vi "initialise_framescan.vi"(8 "error in (no error)":errorcluster) -> (0 "error out":errorcluster, 1 "config cluster":T1={"DDS board initialization parameters"={"Bypass PLL"=FALSE, "PLL Range"=TRUE, "Update Clock"=FALSE, "Triangle "=FALSE, "SDO Active"=FALSE, "LSB First"=FALSE, "OSK Int"=FALSE, "Output Shaped Keying Enable"=TRUE, "Bypass Sinc"=FALSE, "Digital Part"=TRUE, "OutPut DAC"=TRUE, "Control DAC"=TRUE, "Comparator"=FALSE, "Modus"=0, "Multiplier Value"=15}, "OSK select"=TRUE, "inverse?"="normal", "AOD equilibration time"=0.0, "AOD amplitude"=0, "AOD center frequency"=0.0, "AOD Bandwidth"=0.0} {"DDS board initialization parameters"."Modus" scale=0.0..4.0}, 2 "FPGA VI Reference Out":T3, 3 "network streaming queues out":T4)   [LabVIEW 2010]
uses:
  network_streaming_queues_cluster.ctl
  FPGAWrapperMH120124FrameScan_PXI7813R/settings_cluster_framescan.ctl
  common_typedefs/channels_cluster.ctl
  fpgaVIsAndControls/DDS_board_init_cluster.ctl
  fpgaVIsAndControls/gate_cluster.ctl
  common_typedefs/gate_parameters_cluster.ctl
  FPGAWrapperMH120124FrameScan_PXI7813R/configuration_cluster_framescan.ctl
  FPGAWrapperMH120124RAPS_PXI7813R/settings_cluster_raps.ctl
  fpgaVIsAndControls/ellipsoid_parameters_cluster.ctl
  FPGAWrapperMH120124RAPS_PXI7813R/configuration_cluster_raps.ctl
  FPGAWrapperMH120124FrameScan_PXI7813R/FPGA_framescan_reference.ctl
  fpgaVIsAndControls/inverse_enum.ctl
  command_enum.ctl
  <vilib>/userDefined/High Color/nirio_resource_hc.ctl
  <vilib>/rvi/interface/nirviOpenFPGA/nirviOpenFPGA.xnode
  FPGA Bitfiles/FPGA_frame.lvbitx
  <vilib>/rvi/ClientSDK/nirviWhatTheDeviceIsDoing.ctl
  <vilib>/rvi/interface/nirviMethod/nirviMethod.xnode
  <vilib>/rvi/interface/nirviReadWriteControl/nirviReadWriteControl.xnode
  <vilib>/rvi/interface/common/niFpgaNodeNameForErrorReporting.ctl
  <vilib>/rvi/errors/niLvFpgaWhatHappensToTopLevelVI.ctl
  <vilib>/FPGAPlugInAG/PXI-7813R/niLvFpga_Open_PXI-7813R.vi
  <vilib>/rvi/interface/common/dynamic/niFpgaDynamicAddResources.vi
  <vilib>/FPGAPlugInAG/Dynamic/niLvFpga_Reset_Dynamic.vi
  <vilib>/Utility/error.llb/Error Cluster From Error Code.vi
  <vilib>/rvi/errors/niLvFpgaAdjustHostInterfaceError.vi
  NiFpgaLv.dll
panel:
  # "FSK"
  # "Ramped"
  # "FSK"
  # "Chirp Modus"
  # "Unramped"
  # "BPSK"
  # "Single Tone"
  # "FSK"
  # "Ramped"
  # "FSK"
  # "Chirp Modus"
  # "Unramped"
  # "BPSK"
  # "Single Tone"
  # "FSK"
  # "Ramped"
  # "FSK"
  # "Chirp Modus"
  # "Unramped"
  # "BPSK"
  # "Single Tone"
  # "FSK"
  # "Ramped"
  # "FSK"
  # "Chirp Modus"
  # "Unramped"
  # "BPSK"
  # "Single Tone"
  # "FSK"
  # "Ramped"
  # "FSK"
  # "Chirp Modus"
  # "Unramped"
  # "BPSK"
  # "Single Tone"
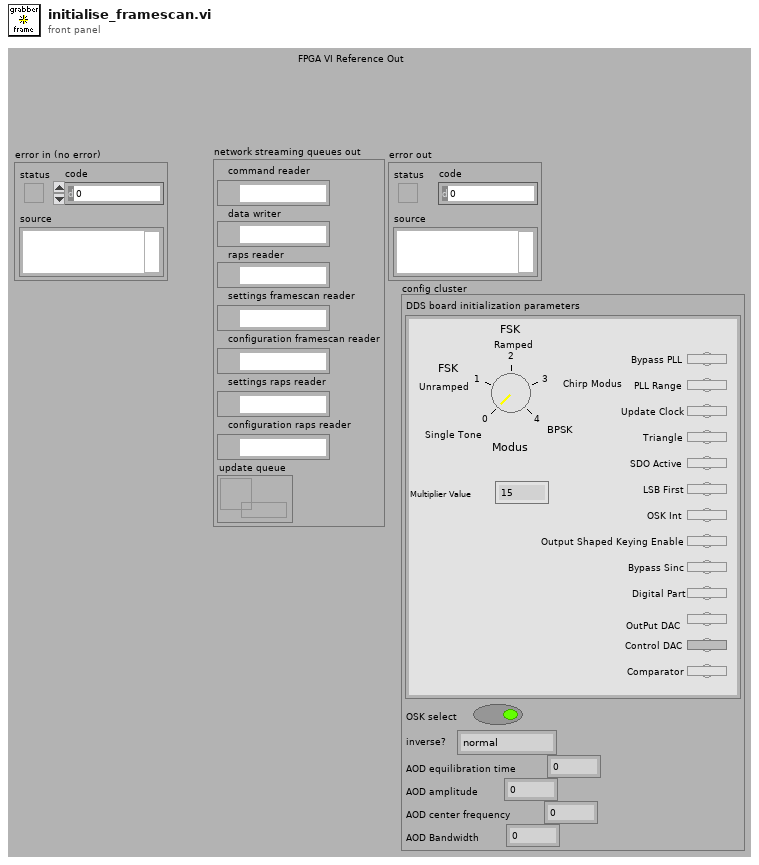
[diagram p1: front panel]
types:
  T1 = typedef "configuration_cluster_framescan.ctl" = cluster{"DDS board initialization parameters":T2, "OSK select":bool, "inverse?":string, "AOD equilibration time":dbl, "AOD amplitude":u16, "AOD center frequency":dbl, "AOD Bandwidth":dbl}
  T2 = typedef "DDS_board_init_cluster.ctl" = cluster{"Bypass PLL":bool, "PLL Range":bool, "Update Clock":bool, "Triangle ":bool, "SDO Active":bool, "LSB First":bool, "OSK Int":bool, "Output Shaped Keying Enable":bool, "Bypass Sinc":bool, "Digital Part":bool, "OutPut DAC":bool, "Control DAC":bool, "Comparator":bool, "Modus":u8, "Multiplier Value":u8}
  T3 = typedef "FPGA_framescan_reference.ctl" = refnum<k20>
  T4 = typedef "network_streaming_queues_cluster.ctl" = cluster{"command reader":refnum<k21>, "data writer":refnum<k21>, "raps reader":refnum<k21>, "settings framescan reader":refnum<k21>, "configuration framescan reader":refnum<k21>, "settings raps reader":refnum<k21>, "configuration raps reader":refnum<k21>, "update queue":refnum<queue>}
  T5 = typedef "inverse_enum.ctl" = enum16{"normal", "x inversed", "y inversed", "x & y inversed"}
  T6 = typedef "command_enum.ctl" = enum8{"NULL", "update", "start", "stop", "reset", "shut-down"}
  T7 = enum32{"Invalid", "Standard", "Closed", "Hidden", "Minimized", "Maximized"}
  T8 = typedef "settings_cluster_framescan.ctl" = cluster{"number of pixels":i32, "iterations per pixel":i32, "maximum bit-depth":i8, "AOD center freq. (Hz)":dbl, "AOD bandwidth freq. (Hz)":dbl, "AOD amplitude":dbl, "pixel dwell time":dbl, "AOD equilibration time":dbl, "x resolution":i32, "y resolution":i32, "z angle (rotation angle, phi)":dbl, "x angle (tilting angle, phi)":dbl, "zoom":dbl, "pixel values cluster":T9, "offset (Hz)":dbl[], "DDS board initialization parameters":T2, "gates":T10[]}
  T9 = typedef "channels_cluster.ctl" = cluster{"channel 0":u32, "channel 1":u32, "channel 2":u32, "channel 3":u32}
  T10 = typedef "gate_cluster.ctl" = cluster{"index":i32, "parameters":T11}
  T11 = typedef "gate_parameters_cluster.ctl" = cluster{"offset":i64, "pulsing":i64, "not pulsing":i64, "cycles per pulse":i64, "repetitions":i64}
  T12 = typedef "nirio_resource_hc.ctl" = tag
  T13 = typedef "niFpgaNodeNameForErrorReporting.ctl" = enum16{"Open FPGA VI Reference", "Read/Write Control", "Invoke Method: Abort", "Invoke Method: Acknowledge IRQ", "Invoke Method: Download", "Invoke Method: FIFO.Configure", "Invoke Method: FIFO.Read", "Invoke Method: FIFO.Start", "Invoke Method: FIFO.Stop", "Invoke Method: FIFO.Write", "Invoke Method: Reset", "Invoke Method: Run", "Invoke Method: Wait on IRQ", "Close FPGA VI Reference"}
  T14 = typedef "niLvFpgaWhatHappensToTopLevelVI.ctl" = enum16{"top level VI scripted behind XNode", "top level VI inlined behind XNode"}
  T15 = cluster{"AOD Bandwidth_x (Hz)":fxp<+/-,36,32>, "AOD Bandwidth_y (Hz)":fxp<+/-,36,32>, "sin Phi":fxp<+/-,36,2>, "cos Phi":fxp<+/-,36,2>, "Bandwidth for LUTs (256pts)":fxp<+,36,0>, "AOD_Amplitude in":u16, "AOD center frequ. (Hz)_x":fxp<+/-,36,32>, "AOD center frequ. (Hz)_y":fxp<+/-,36,32>, "x offset (Hz)":fxp<+/-,36,32>, "y offset (Hz)":fxp<+/-,36,32>}
  T16 = typedef "nirviWhatTheDeviceIsDoing.ctl" = enum32{"nothing", "something other than LabVIEW FPGA", "FPGA interface", "interactive", "emulation"}
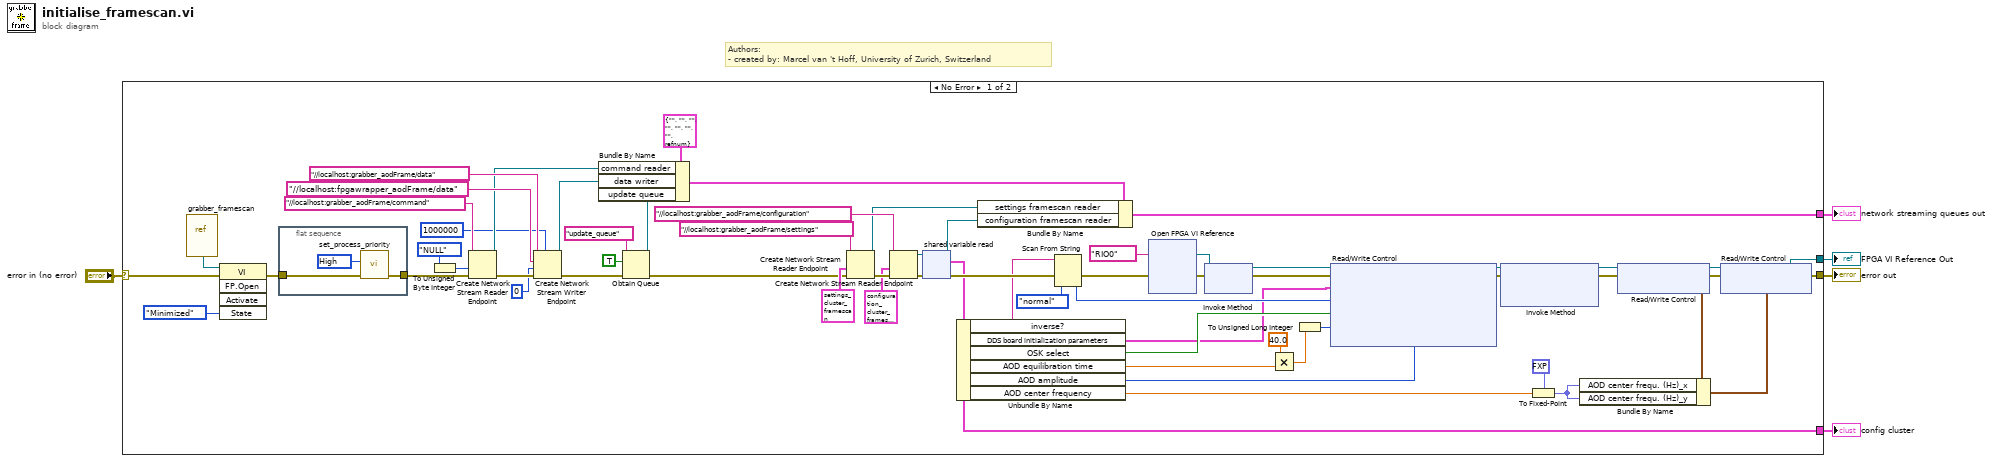
[diagram p0: block diagram]
diagram:
  # "Authors: \n- created by: Marcel van 't Hoff, University of Zurich, Switzerland"
  n1 = case shown="No Error" "error in (no error)" {
    selector: "error in (no error)" -> [w54 w397]
    tunnel: [w57 _] -> w5
    tunnel: [w38 w397] -> w4
    tunnel: [w40 _] -> w2
    tunnel: [w6 _] -> w1
    frame No Error {
      n2 = vi-ref "grabber_framescan.vi"() -> (w52:refnum<vi>)
      n3 = invoke class="VI" method="FP.Open"(reference=w52, error in=w54, "State"=T7."Minimized") -> (error out=w35:errorcluster)  [unwired: 2 in, 4 out]
      n4 = flat-sequence {
        tunnel: w35 -> [w71]
        tunnel: [w70] -> w19
        frame #0 {
          w69 = 128 items=["Normal"=32, "Idle"=64, "High"=128, "RealTime"=256, "BelowNormal"=16384, "AboveNormal"=32768] ("PriorityClass")
          n5 = call "set_process_priority.vi"("error in (no error)"=w71, "PriorityClass"=w69) -> ("error out"=w70:errorcluster)  [unwired: 9 in]
        }
      }
      n6 = To Unsigned Byte Integer(number=command_enum."NULL" ("command")) -> (unsigned 8bit integer=w30:u8)
      n7 = Create Network Stream Reader Endpoint(8:w19, 9:w30, 11:"//localhost:grabber_aodFrame/command" ("writer name")) -> (0:w29:errorcluster, 3:w24:refnum<k21>)  [unwired: 3 in]
      n8 = Create Network Stream Writer Endpoint(5:1000000 ("writer buffer size"), 8:w29, 9:u64 0, 10:"//localhost:fpgawrapper_aodFrame/data" ("reader url"), 11:"//localhost:grabber_aodFrame/data" ("writer name")) -> (0:w15:errorcluster, 3:w14:refnum<k21>)  [unwired: 1 in]
      n9 = Obtain Queue(name (unnamed)="update_queue", element data type=TRUE, error in (no error)=w15) -> (queue out=w20:refnum<queue>, error out=w34:errorcluster)  [unwired: 2 in, 1 out]
      n10 = Bundle By Name(cluster=T4 {"command reader"="", "data writer"="", "raps reader"="", "settings framescan reader"="", "configuration framescan reader"="", "settings raps reader"="", "configuration raps reader"="", "update queue"=refnum} ("network streaming queues"), "command reader"=w24, "data writer"=w14, "update queue"=w20) -> (w33:T4)
      n11 = Create Network Stream Reader Endpoint(8:w34, 9:T8 {"number of pixels"=0, "iterations per pixel"=0, "maximum bit-depth"=0, "AOD center freq. (Hz)"=0.0, "AOD bandwidth freq. (Hz)"=0.0, "AOD amplitude"=0.0, "pixel dwell time"=0.0, "AOD equilibration time"=0.0, "x resolution"=0, "y resolution"=0, "z angle (rotation angle, phi)"=0.0, "x angle (tilting angle, phi)"=0.0, "zoom"=0.0, "pixel values cluster"={"channel 0"=0, "channel 1"=0, "channel 2"=0, "channel 3"=0}, "offset (Hz)"=[], "DDS board initialization parameters"={"Bypass PLL"=FALSE, "PLL Range"=FALSE, "Update Clock"=FALSE, "Triangle "=FALSE, "SDO Active"=FALSE, "LSB First"=FALSE, "OSK Int"=FALSE, "Output Shaped Keying Enable"=FALSE, "Bypass Sinc"=FALSE, "Digital Part"=FALSE, "OutPut DAC"=FALSE, "Control DAC"=FALSE, "Comparator"=FALSE, "Modus"=0, "Multiplier Value"=0}, "gates"=[]} ("settings cluster"), 11:"//localhost:grabber_aodFrame/settings" ("reader name")) -> (0:w66:errorcluster, 3:w55:refnum<k21>)  [unwired: 3 in]
      n12 = Create Network Stream Reader Endpoint(8:w66, 9:T1 {"DDS board initialization parameters"={"Bypass PLL"=FALSE, "PLL Range"=FALSE, "Update Clock"=FALSE, "Triangle "=FALSE, "SDO Active"=FALSE, "LSB First"=FALSE, "OSK Int"=FALSE, "Output Shaped Keying Enable"=FALSE, "Bypass Sinc"=FALSE, "Digital Part"=FALSE, "OutPut DAC"=FALSE, "Control DAC"=FALSE, "Comparator"=FALSE, "Modus"=0, "Multiplier Value"=0}, "OSK select"=FALSE, "inverse?"="normal", "AOD equilibration time"=0.0, "AOD amplitude"=0, "AOD center frequency"=0.0, "AOD Bandwidth"=0.0} ("config cluster"), 11:"//localhost:grabber_aodFrame/configuration" ("reader name")) -> (0:w65:errorcluster, 3:w64:refnum<k21>)  [unwired: 3 in]
      n13 = shared-variable-read(w64, w65) -> (w46:refnum<k21>, w49:errorcluster, w6:T1)  [unwired: 1 in, 1 out]
      n14 = Unbundle By Name(w6) -> ("inverse?"=w47:string, "DDS board initialization parameters"=w7:T2, "OSK select"=w11:bool, "AOD equilibration time"=w17:dbl, "AOD amplitude"=w10:u16, "AOD center frequency"=w16:dbl)
      n15 = Bundle By Name(cluster=w33, "settings framescan reader"=w55, "configuration framescan reader"=w46) -> (w57:T4)
      n16 = Scan From String(input string=w47, error in=w49, default 1=inverse_enum."normal" ("inverse?")) -> (error out=w48:errorcluster, output 1=w13:T5)  [unwired: 2 in, 2 out]
      n17 = xnode "Open FPGA VI Reference"("error in"=w48, "resource name"=T12 "RIO0") -> ("FPGA VI Reference Out"=w68:refnum<k20>, "error out"=w67:errorcluster)
      n18 = xnode "Invoke Method"("FPGA VI Reference In"=w68, "error in"=w67) -> ("FPGA VI Reference Out"=w63:refnum<k20>, "error out"=w62:errorcluster)
      n19 = Multiply(x=40.0, y=w17) -> (x*y=w45:dbl)
      n20 = To Unsigned Long Integer(number=w45) -> (unsigned 32bit integer=w12:u32)
      n21 = xnode "Read/Write Control"("FPGA VI Reference In"=w63, "error in"=w62, "DDS board initialization parameters"=w7, "inverse?"=w13, "OSK select"=w11, "waiting iterations  per pixel"=w12, "amplitude"=w10) -> ("FPGA VI Reference Out"=w51:refnum<k20>, "error out"=w61:errorcluster)
      n22 = xnode "Invoke Method"("FPGA VI Reference In"=w51, "error in"=w61) -> ("FPGA VI Reference Out"=w43:refnum<k20>, "error out"=w42:errorcluster)  [unwired: 1 in]
      n23 = To Fixed-Point(fixed-point type=fxp<+/-,36,32> 0.0 ("AOD center frequ. (MHz)"), number=w16) -> (fixed-point=w37:fxp<+/-,36,32>)
      n24 = xnode "Read/Write Control"("FPGA VI Reference In"=w43, "error in"=w42) -> ("FPGA VI Reference Out"=w41:refnum<k20>, "error out"=w39:errorcluster, "FPGA parameters"=w9:T15)
      n25 = Bundle By Name(cluster=w9, "AOD center frequ. (Hz)_x"=w37, "AOD center frequ. (Hz)_y"=w37) -> (w8:T15)
      n26 = xnode "Read/Write Control"("FPGA VI Reference In"=w41, "error in"=w39, "FPGA parameters"=w8) -> ("FPGA VI Reference Out"=w40:refnum<k20>, "error out"=w38:errorcluster)
    }
    frame Error {
    }
  }
  "network streaming queues out" <- w5
  "error out" <- w4
  "FPGA VI Reference Out" <- w2
  "config cluster" <- w1
